vi "FormEnsaio.vi"() -> ()   [LabVIEW 2014]
panel:
  out "Velocidde (Km/h)":dbl(knob) scale=0.0..150.0
  out "Velocidade Inferior":string
  out "labelUpperSpeed":string caption="Velocidade Superior"
  out "gaugeForca":dbl(knob) caption="Força (Kgf)" scale=0.0..100.0
  in  "Ciclo 2":dbl(slide) scale=0.0..10.0
  in  "Ciclo 1":dbl(slide) scale=0.0..10.0
  out "Rotação (RPM)":dbl(knob) scale=0.0..800.0
  out "Termopar B":dbl[unit](slide)=273.15 scale=273.15..973.15
  out "Termopar A":dbl[unit](slide)=273.15 scale=273.15..973.15
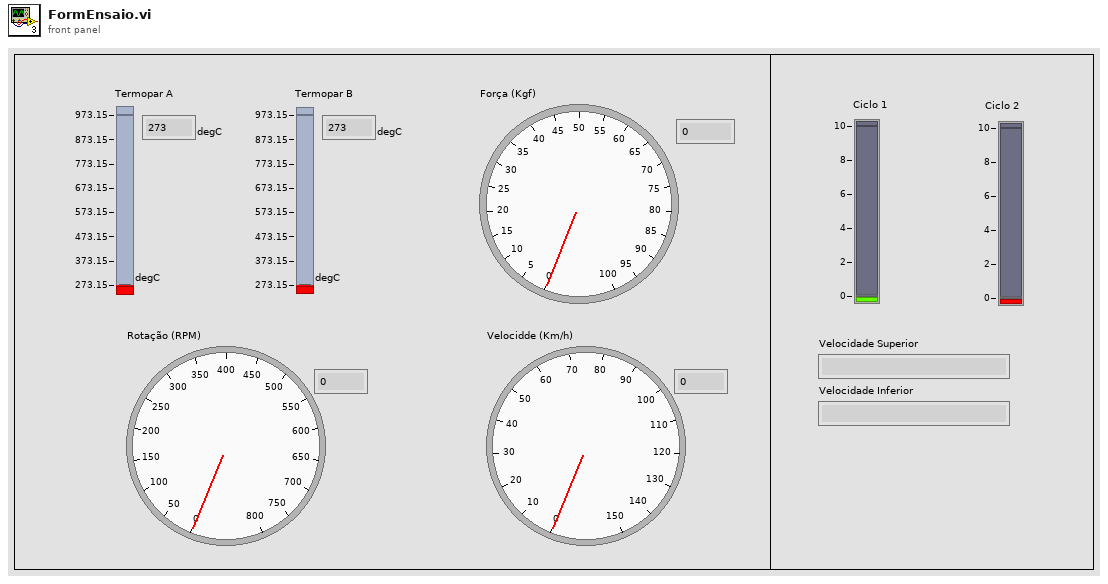
[diagram p1: front panel]
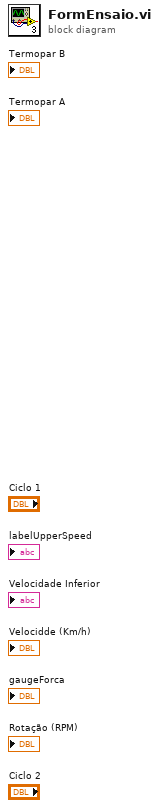
[diagram p0: block diagram]
diagram:
